vi "Grab Stamp.vi"(8 "error in":errorcluster, 10 "Stamp Number":i32, 11 "GrabberTool in":refnum<class "GrabberTool Class.lvclass">) -> (0 "error out":errorcluster, 3 "GrabberTool out":refnum<class "GrabberTool Class.lvclass">)   [LabVIEW 2011, in "GrabberTool Class.lvclass"]
uses:
  GrabberTool Class.lvclass
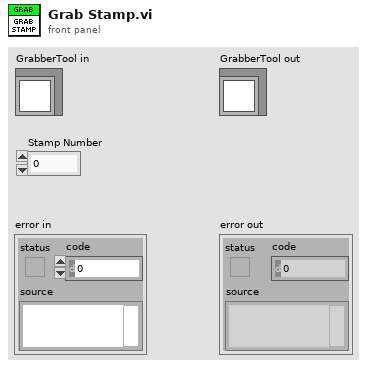
[diagram p1: front panel]
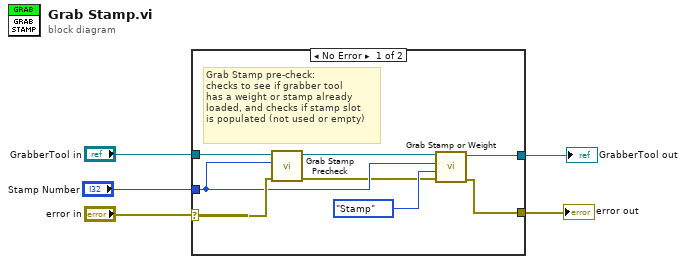
[diagram p0: block diagram]
diagram:
  n1 = case shown="No Error" "error in" {
    selector: "error in" -> [w12 w14]
    tunnel: "GrabberTool in" -> [w13 w15]
    tunnel: "Stamp Number" -> [w10 _]
    tunnel: [w6 w15] -> w2
    tunnel: [w7 w14] -> w1
    frame No Error {
      # "Grab Stamp pre-check:\nchecks to see if grabber tool\nhas a weight or stamp already \nloaded, and checks if stamp slot\nis populated (not used or empty)"
      n2 = call "Grab Stamp Precheck.vi"("error in (no error)"=w12, "Stamp Number"=w10, "GrabberTool Class in"=w13) -> ("error out"=w8:errorcluster, "GrabberTool Class out"=w11:refnum<class "GrabberTool Class.lvclass">)  [unwired: 7 in]
      n3 = call "Grab Stamp or Weight.vi"("error in"=w8, "Tool Type"=enum16{"Stamp", "Weight"}."Stamp", "Slot Number"=w10, "GrabberTool in"=w11) -> ("error out"=w7:errorcluster, "GrabberTool out"=w6:refnum<class "GrabberTool Class.lvclass">)  [unwired: 6 in]
    }
    frame Error {
    }
  }
  "GrabberTool out" <- w2
  "error out" <- w1
